vi "DIMPowerSupply.ConvertControl.vi"(0 "i ref in":refnum<vi>, 2 "nominal PS voltage [V]":dbl format="%.2f", 5 "error in (no error)":errorcluster) -> (14 "i ref out":refnum<vi>, 16 "nominal module value":dbl, 18 "nominal module voltage [V]":dbl format="%.2f", 19 "error out":errorcluster)   [LabVIEW 2014, in "DIMPowerSupply.lvlib"]
doc: "Converts the nominal voltage value [V] of the power supply to 1) the voltage of the module (controlling the analog input of the power supply) and 2) the (integer)set-value of the module."
uses:
  DIMPowerSupply.lvlib
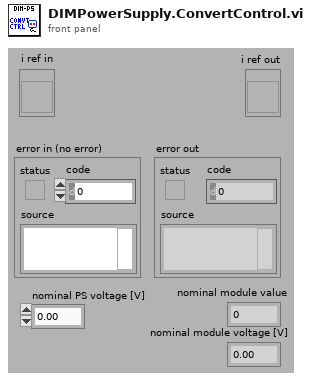
[diagram p1: front panel]
types:
  T1 = typedef "DIMPowerSupply.lvlib/DIMPowerSupply.ranges type.ctl" = cluster{"deviceMin":dbl, "deviceMax":dbl, "numberMin":u16, "numberMax":u16, "U16?":bool, "factor":dbl}
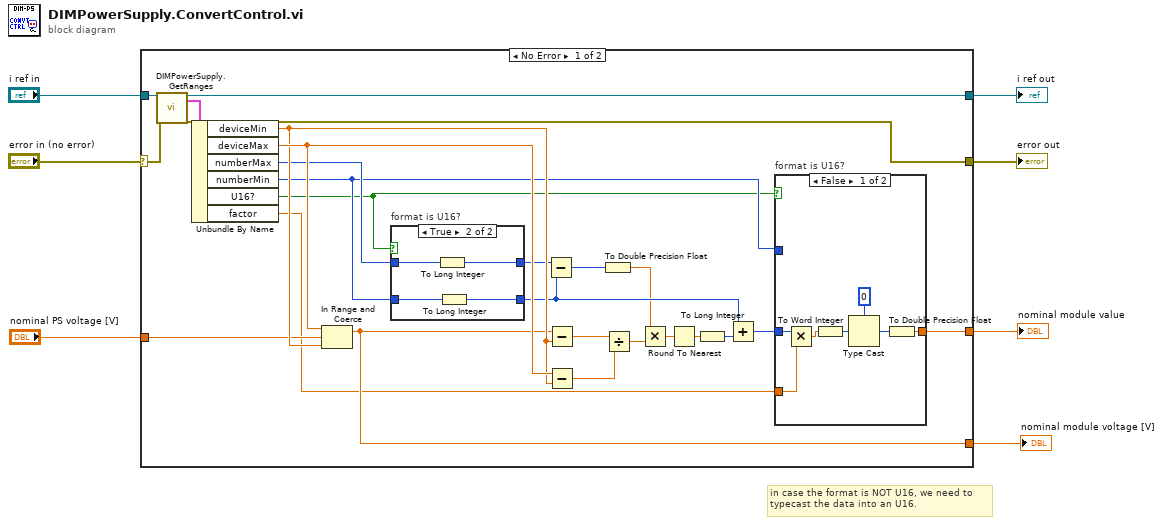
[diagram p0: block diagram]
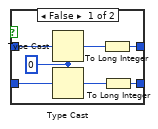
[diagram p2: hidden frame]
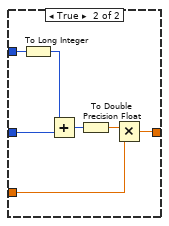
[diagram p3: hidden frame]
diagram:
  # "in case the format is NOT U16, we need to\ntypecast the data into an U16."
  n1 = case shown="No Error" "error in (no error)" {
    selector: "error in (no error)" -> [w24 w58]
    tunnel: "i ref in" -> [w31 w59]
    tunnel: [w30 w59] -> w6
    tunnel: [w29 w58] -> w5
    tunnel: [w8 _] -> w4
    tunnel: "nominal PS voltage [V]" -> [w26 _]
    tunnel: [w25 _] -> w2
    frame No Error {
      n2 = call "DIMPowerSupply.GetRanges.vi"("i ref in"=w31, "error in (no error)"=w24) -> ("i ref out"=w30:refnum<vi>, "ControlRanges"=w32:T1, "error out"=w29:errorcluster)  [unwired: 14 in, 1 out]
      n3 = Unbundle By Name(w32) -> ("deviceMin"=w27:dbl, "deviceMax"=w28:dbl, "numberMax"=w23:u16, "numberMin"=w13:u16, "U16?"=w12:bool, "factor"=w9:dbl)
      n4 = In Range and Coerce(upper limit=w28, x=w26, lower limit=w27) -> (coerced(x)=w25:dbl)  [unwired: 1 out]
      n5 = case "format is U16?" shown="True" w12 {
        tunnel: w23 -> [w39 w43]
        tunnel: [w36 w42] -> w19
        tunnel: [w35 w40] -> w15
        tunnel: w13 -> [w34 w41]
        frame False {
          w33 = i16 0
          n6 = Type Cast(type=w33, x=w39) -> (*(type *) &x=w38:i16)
          n7 = Type Cast(type=w33, x=w34) -> (*(type *) &x=w37:i16)
          n8 = To Long Integer(number=w38) -> (32bit integer=w36:i32)
          n9 = To Long Integer(number=w37) -> (32bit integer=w35:i32)
        }
        frame True {
          n10 = To Long Integer(number=w43) -> (32bit integer=w42:i32)
          n11 = To Long Integer(number=w41) -> (32bit integer=w40:i32)
        }
      }
      n12 = Subtract(x=w19, y=w15) -> (x-y=w17:i32)
      n13 = Subtract(x=w25, y=w27) -> (x-y=w18:dbl)
      n14 = Subtract(x=w28, y=w27) -> (x-y=w22:dbl)
      n15 = To Double Precision Float(number=w17) -> (double precision float=w14:dbl)
      n16 = Divide(x=w18, y=w22) -> (x/y=w21:dbl)
      n17 = Multiply(x=w14, y=w21) -> (x*y=w20:dbl)
      n18 = Round To Nearest(number=w20) -> (nearest integer value=w16:dbl)
      n19 = To Long Integer(number=w16) -> (32bit integer=w10:i32)
      n20 = Add(x=w15, y=w10) -> (x+y=w11:i32)
      n21 = case "format is U16?" shown="False" w12 {
        tunnel: w11 -> [w46 w57]
        tunnel: w13 -> [_ w56]
        tunnel: [w47 w52] -> w8
        tunnel: w9 -> [w45 w51]
        frame False {
          n22 = Multiply(x=w46, y=w45) -> (x*y=w44:dbl)
          n23 = To Word Integer(number=w44) -> (16bit integer=w50:i16)
          n24 = Type Cast(type=u16 0, x=w50) -> (*(type *) &x=w48:u16)
          n25 = To Double Precision Float(number=w48) -> (double precision float=w47:dbl)
        }
        frame True {
          n26 = To Long Integer(number=w56) -> (32bit integer=w55:i32)
          n27 = Add(x=w55, y=w57) -> (x+y=w53:i32)
          n28 = To Double Precision Float(number=w53) -> (double precision float=w54:dbl)
          n29 = Multiply(x=w54, y=w51) -> (x*y=w52:dbl)
        }
      }
    }
    frame Error {
    }
  }
  "error out" <- w5
  "i ref out" <- w6
  "nominal module value" <- w4
  "nominal module voltage [V]" <- w2
